vi "Speichern.vi"(8 "Fehler (Eingang)":errorcluster caption="Fehler (Ausgang)", 11 "pfad":path) -> (0 "Fehler (Ausgang)":errorcluster)   [LabVIEW 2020, in "FT-IR.lvlib" / "Spanfaktor.lvlib"]
uses:
  Spanfaktor.lvlib
  Aktion FGV Span.ctl
  FGV FT-IR Aktionen.ctl
  FGV FT-IR Gasliste Aktionen.ctl
  Aktionen EVID-Codes.ctl
  System Einstellungen V2/Aktioen FGV System Konstanten.ctl
  FT-IR.lvlib
  System Einstellungen V2/System Einstellungen V2.lvlib
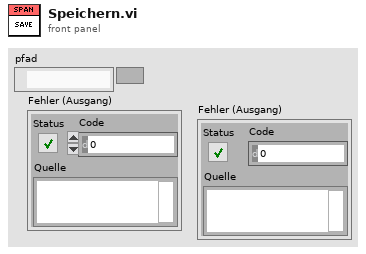
[diagram p1: front panel]
types:
  T1 = typedef "System Einstellungen V2.lvlib/Aktioen FGV System Konstanten.ctl" = enum16{"lesen", "laden", "speichern", "Sprache"}
  T2 = typedef "FT-IR.lvlib/Aktionen EVID-Codes.ctl" = enum16{"lesen", "setzen", "laden", "speichern", "1Hz/5Hz", "Smoothing", "Rolling Average"}
  T3 = typedef "FT-IR.lvlib/FGV FT-IR Gasliste Aktionen.ctl" = enum16{"lesen", "Gasliste FT-IR", "Gasliste ausgelesen", "laden", "speichern", "löschen"}
  T4 = typedef "FT-IR.lvlib/FGV FT-IR Aktionen.ctl" = enum16{"lesen", "NOG setzen", "NOS setzen", "Initialisieren", "speichern", "ALLES setzen", "FT-IR Spektrum loggen", "Komm Stoppen", "Spektrum LogKonfig"}
  T5 = enum16{"open", "replace", "create", "open or create", "replace or create", "replace or create with confirmation"}
  T6 = typedef "FT-IR.lvlib/Spanfaktor.lvlib/Aktion FGV Span.ctl" = enum16{"lesen", "Span", "Seite aktiv", "Offset", "FGV aktualisiert", "Aktualisierung aufheben"}
  T7 = cluster{"Modell":string, "ProjektNummer":string, "Software Version":string, "Seriennummer":string}
  T8 = typedef "String - Ausgabefeld.ctl" = string
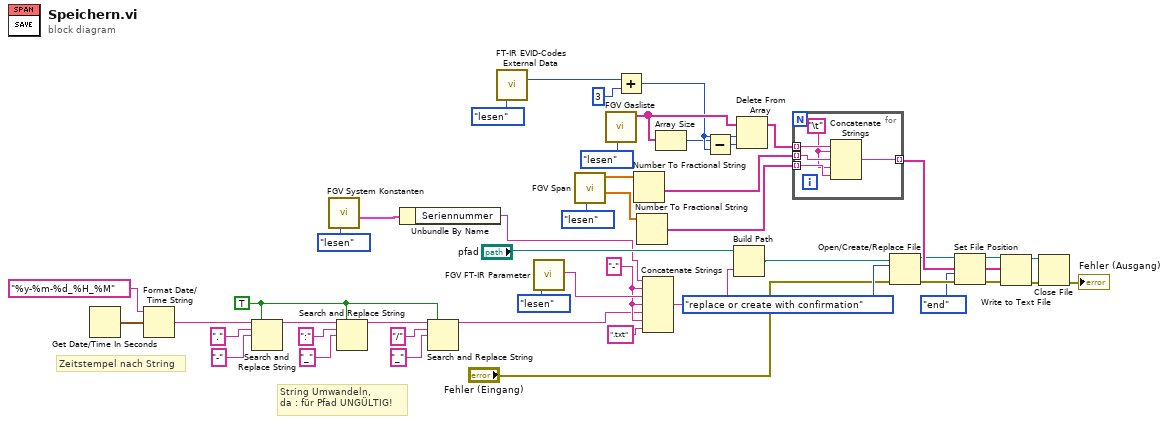
[diagram p0: block diagram]
diagram:
  w7 = TRUE ("Alle ersetzen? (F)")
  w5 = "-" ("String")
  # "String Umwandeln, \nda : für Pfad UNGÜLTIG!"
  # "Zeitstempel nach String"
  n1 = Get Date/Time In Seconds() -> (seconds since 1Jan1904=w17:timestamp)
  n2 = Format Date/Time String(time format string (%c)="%y-%m-%d_%H_%M" ("Zeitformatierungs-String (%c)"), seconds (now)=w17) -> (date/time string=w16:string)  [unwired: 1 in]
  n3 = Search and Replace String(replace all?=w7, input string=w16, search string="." ("Such-String"), replace string="-" ("String ersetzen(\"\")")) -> (result string=w13:string)  [unwired: 4 in, 3 out]
  n4 = call "FGV System Konstanten.vi"("Aktionen"=Aktioen_FGV_System_Konstanten."lesen") -> ("Cluster out"=w1:T7)  [unwired: 6 in, 4 out]
  n5 = Search and Replace String(replace all?=w7, input string=w13, search string=":" ("Such-String"), replace string="_" ("String ersetzen(\"\")")) -> (result string=w8:string)  [unwired: 4 in, 3 out]
  n6 = Unbundle By Name(w1) -> ("Seriennummer"=w3:string)
  n7 = Search and Replace String(replace all?=w7, input string=w8, search string="/" ("Such-String"), replace string="_" ("String ersetzen(\"\")")) -> (result string=w4:string)  [unwired: 4 in, 3 out]
  n8 = call "FT-IR EVID-Codes External Data.vi"("Aktionen"=Aktionen_EVID-Codes."lesen") -> ("Anzahl"=w45:i32)  [unwired: 9 in, 5 out]
  n9 = call "FGV FT-IR Parameter.vi"("Aktion"=FGV_FT-IR_Aktionen."lesen") -> ("Current Recipe"=w23:string)  [unwired: 11 in, 7 out]
  n10 = call "FGV Span.vi"("Aktion"=Aktion_FGV_Span."lesen") -> ("Offset"=w26:sgl[], "Span"=w25:sgl[])  [unwired: 7 in, 2 out]
  n11 = call "FGV Gasliste.vi"("Aktionen"=FGV_FT-IR_Gasliste_Aktionen."lesen") -> ("Aktuelle Gasliste FT-IR"=w43:T8[])  [unwired: 8 in, 2 out]
  n12 = Add(x=w45, y=3) -> (x+y=w42:i32)
  n13 = Number To Fractional String(number=w25) -> (F-format string=w36:string[])  [unwired: 3 in]
  n14 = Number To Fractional String(number=w26) -> (F-format string=w37:string[])  [unwired: 3 in]
  n15 = Concatenate Strings(w3, w5, w23, w5, w4, w5, ".txt" ("String")) -> (w18:string)
  n16 = Array Size(array=w43) -> (size(s)=w41:i32)
  n17 = Subtract(x=w41, y=w42) -> (x-y=w40:i32)
  n18 = Build Path(base path="pfad", name or relative path=w18) -> (appended path=w22:path)
  n19 = Delete From Array(array=w43, length=w42, index=w40) -> (array with subset deleted=w48:T8[])  [unwired: 1 out]
  n20 = for {
    tunnel: w48 -> [w53] mode=indexing
    tunnel: w36 -> [w52] mode=indexing
    tunnel: w37 -> [w51] mode=indexing
    tunnel: [w49] -> w38 mode=indexing
    w50 = "\t"
    n21 = Concatenate Strings(w53, w50, w52, w50, w51) -> (w49:string)
  }
  n22 = Open/Create/Replace File(file path (use dialog)=w22, error in="Fehler (Eingang)", operation (0:open)=T5."replace or create with confirmation" ("Operation (0:Öffnen)")) -> (refnum out=w32:refnum<file>, error out=w31:errorcluster)  [unwired: 3 in, 1 out]
  n23 = Set File Position(refnum=w32, from (0:start)=enum16{"start", "end", "current"}."end" ("Von (0:Start)"), error in=w31) -> (refnum out=w33:refnum<file>, error out=w34:errorcluster)  [unwired: 1 in]
  n24 = Write to Text File(file (use dialog)=w33, text=w38, error in=w34) -> (refnum out=w28:refnum<file>, error out=w27:errorcluster)  [unwired: 1 in, 1 out]
  n25 = Close File(refnum=w28, error in=w27) -> (error out=→"Fehler (Ausgang)":errorcluster)  [unwired: 1 out]
